vi "Generate Temporary Class Path.vi"(8 "error in (no error)":errorcluster) -> (0 "error out":errorcluster, 3 "appended path":path)   [LabVIEW 2020, in "Mock Class Updater.lvclass"]
uses:
  Mock Class Updater.lvclass
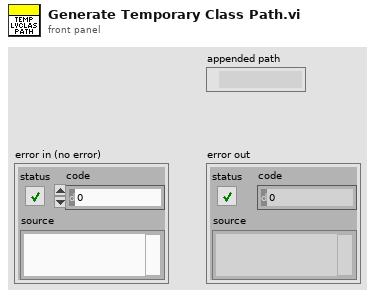
[diagram p1: front panel]
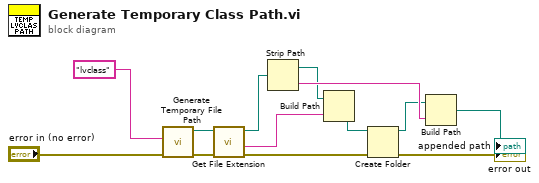
[diagram p0: block diagram]
diagram:
  n1 = call <vilib>:"Generate Temporary File Path.vi"("error in (no error)"="error in (no error)", "Temporary File Extension (tmp)"="lvclass") -> ("error out"=w2:errorcluster, "Unique Temporary File Path"=w5:path)  [unwired: 8 in]
  n2 = call <vilib>:"Get File Extension.vi"("error in (no error)"=w2, "file"=w5) -> ("error out"=w4:errorcluster, "filename without extension"=w8:string, "dup file"=w6:path)  [unwired: 5 in, 2 out]
  n3 = Strip Path(path=w6) -> (stripped path=w7:path, name=w12:string)
  n4 = Build Path(base path=w7, name or relative path=w8) -> (appended path=w10:path)
  n5 = Create Folder(path (use dialog)=w10, error in=w4) -> (created path=w11:path, error out=→"error out":errorcluster)  [unwired: 1 in, 1 out]
  n6 = Build Path(base path=w11, name or relative path=w12) -> (appended path=→"appended path":path)
